vi "Get Measure.vi"(8 "error in (no error)":errorcluster caption="entrée d'erreur (pas d'erreur)", 11 "Class LED Analyser in":refnum<class "Class LED Analyser FEASA.lvclass">) -> (0 "error out":errorcluster caption="sortie d'erreur", 3 "Class LED Analyser Out":refnum<class "Class LED Analyser FEASA.lvclass">)   [LabVIEW 2020, in "Library Instrument & Equipement.lvlib" / "Library LED Analyser.lvlib" / "Class LED Analyser FEASA.lvclass"]
uses:
  Class LED Analyser FEASA.lvclass
  C:/Users/ngarcin/OneDrive - Altyor/Standard TB/Class/LED Analyser/Class Led Analyser (Default)/Class LED Analyser (Default).lvclass
  Class LED Analyser FEASA.lvclass/Class LED Analyser FEASA.ctl
  LED Analyser/Library LED Analyser.lvlib
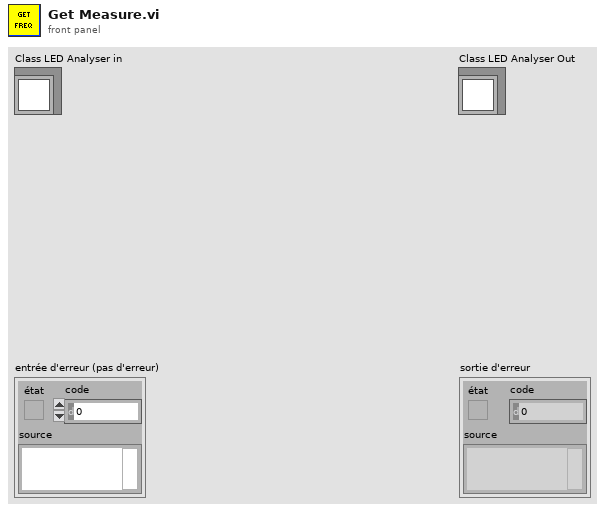
[diagram p1: front panel]
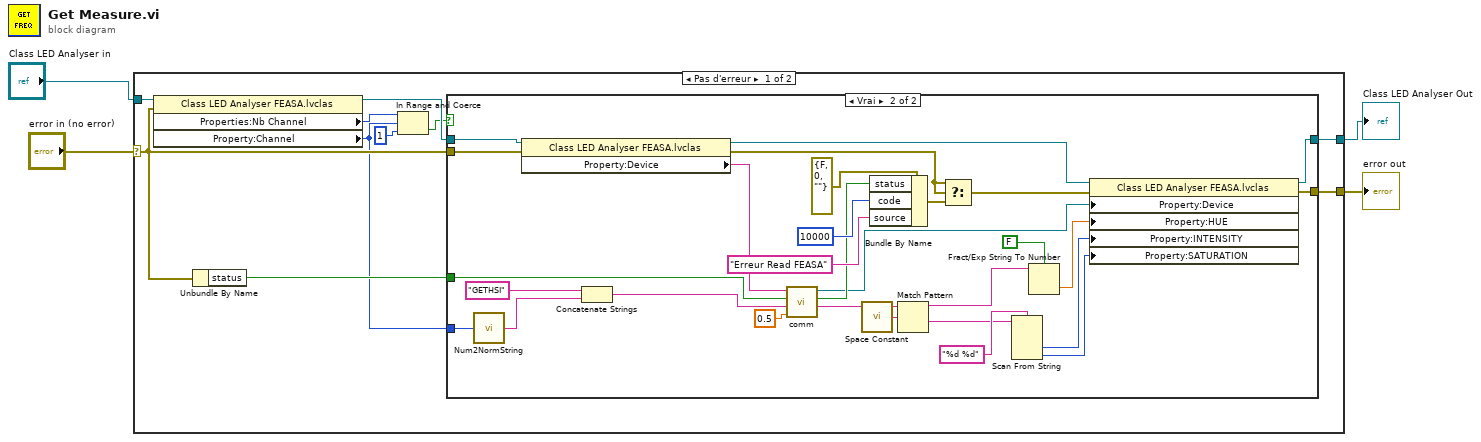
[diagram p0: block diagram]
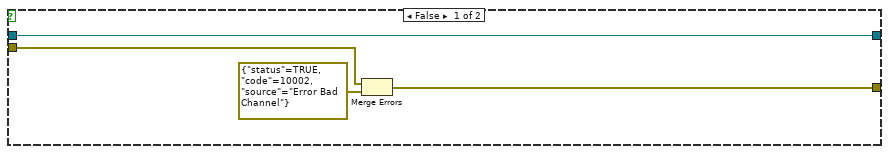
[diagram p2: hidden frame]
diagram:
  n1 = case shown="Pas d'erreur" "error in (no error)" {
    selector: "error in (no error)" -> [w12 w49]
    tunnel: [w10 w49] -> w3
    tunnel: [w11 w48] -> w1
    tunnel: "Class LED Analyser in" -> [w13 w48]
    frame No Error {
      n2 = property class="Class LED Analyser FEASA.lvclas"(reference=w13, error in=w12) -> (reference out=w9:refnum<class "Class LED Analyser FEASA.lvclass">, "Properties:Nb Channel"=w5:u16, "Property:Channel"=w8:u16)  [unwired: 1 out]
      n3 = Unbundle By Name(w12) -> ("status"=w14:bool)
      n4 = In Range and Coerce(upper limit=w5, x=w8, lower limit=u16 1 ("limite inférieure")) -> (In Range?=w6:bool)  [unwired: 1 out]
      n5 = case shown="Vrai" w6 {
        tunnel: w14 -> [_ w43]
        tunnel: w12 -> [w15 w31]
        tunnel: [w18 w36] -> w11
        tunnel: [w16 w34] -> w10
        tunnel: w9 -> [w18 w32]
        tunnel: w8 -> [_ w33]
        frame False {
          n6 = Merge Errors(w15, errorcluster {"status"=TRUE, "code"=10002, "source"="Error Bad Channel"} ("error IO")) -> (w16:errorcluster)
        }
        frame True {
          n7 = call "Num2NormString.vi"("Number"=w33) -> ("Normalized String Number"=w46:string)
          n8 = property class="Class LED Analyser FEASA.lvclas"(reference=w32, error in=w31) -> (reference out=w27:refnum<class "Class LED Analyser FEASA.lvclass">, error out=w30:errorcluster, "Property:Device"=w29:string)
          n9 = Concatenate Strings("GETHSI" ("Command"), w46) -> (w45:string)
          n10 = call "comm.vi"("Timeout (s)"=0.5, "Command"=w45, "Error"=w43, "VISA resource name"=w29) -> ("Response"=w26:string, "Error"=w38:bool, "dup VISA resource name"=w28:refnum<visa-resource-name>)  [unwired: 2 in, 1 out]
          n11 = call <vilib>:"Space Constant.vi"() -> ("String"=w25:string)
          n12 = Bundle By Name(cluster=errorcluster {"status"=FALSE, "code"=0, "source"=""} ("error IO"), "status"=w38, "code"=10000, "source"="Erreur Read FEASA") -> (w39:errorcluster)
          n13 = Match Pattern(string=w26, regular expression=w25) -> (before substring=w24:string, after substring=w19:string)  [unwired: 1 in, 2 out]
          n14 = Select(t=w30, s=w30, f=w39) -> (s? t:f=w35:errorcluster)
          n15 = Scan From String(format string="%d %d", input string=w19) -> (output 1=w22:i32, output 2=w21:i32)  [unwired: 4 in, 3 out]
          n16 = Fract/Exp String To Number(use system decimal point (T)=FALSE, string=w24) -> (number=w20:dbl)  [unwired: 2 in, 1 out]
          n17 = property class="Class LED Analyser FEASA.lvclas"(reference=w27, error in=w35, "Property:Device"=w28, "Property:HUE"=w20, "Property:INTENSITY"=w22, "Property:SATURATION"=w21) -> (reference out=w36:refnum<class "Class LED Analyser FEASA.lvclass">, error out=w34:errorcluster)
        }
      }
    }
    frame Error {
    }
  }
  "error out" <- w3
  "Class LED Analyser Out" <- w1
